vi "GetObjectConfigurationString.vi"(8 "ErrorIn":errorcluster, 10 "Label":string, 11 "ReferenceIn":refnum<class "AppConfigJSON.lvclass">) -> (0 "ErrorOut":errorcluster, 1 "String":string, 2 "Identification":string, 3 "ReferenceOut":refnum<class "AppConfigJSON.lvclass">)   [LabVIEW 2021, in "AppConfigJSON.lvclass"]
uses:
  AppConfigJSON.lvclass
  AppConfigJSON.lvclass/AppConfigJSON.ctl
  <vilib>/JDP Science/JSONtext/Config Files/Config File.lvclass
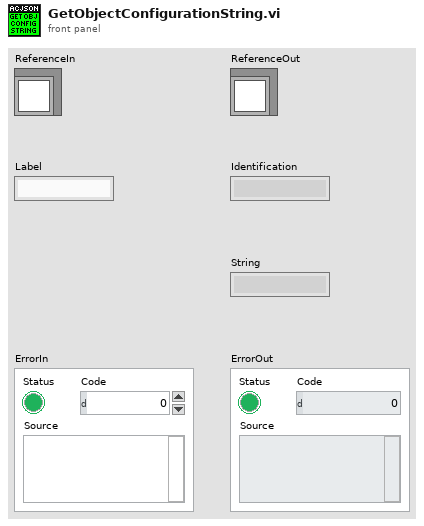
[diagram p1: front panel]
types:
  T1 = typedef "AppConfigJSON.lvclass/ObjectAttributes.ctl" = cluster{"Name":string, "ConfigFilePath":path, "Objects":T2[], "ApplicationBasePath":path, "ObjectName":string}
  T2 = typedef "IApplicationConfiguration.lvclass/ObjectDataDetails.ctl" = cluster{"ObjectName":string, "ObjectType":string, "Interfaces":T3[]}
  T3 = typedef "IApplicationConfiguration.lvclass/ObjectData.ctl" = cluster{"Label":string, "ObjectName":string, "Type":string}
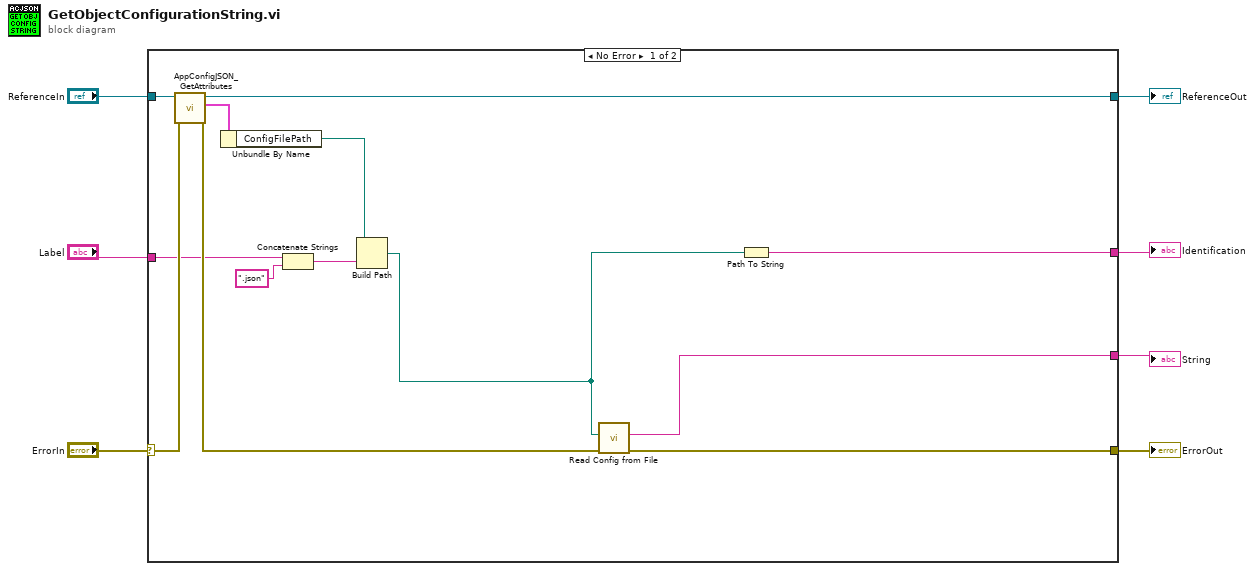
[diagram p0: block diagram]
diagram:
  n1 = case shown="No Error" "ErrorIn" {
    selector: "ErrorIn" -> [w19 w21]
    tunnel: [w18 w21] -> w6
    tunnel: [w15 w20] -> w4
    tunnel: "ReferenceIn" -> [w16 w20]
    tunnel: "Label" -> [w11 _]
    tunnel: [w10 _] -> w2
    tunnel: [w8 _] -> w1
    frame No Error {
      n2 = call "AppConfigJSON_GetAttributes.vi"("ErrorIn"=w19, "ReferenceIn"=w16) -> ("ErrorOut"=w18:errorcluster, "Data"=w17:T1, "ReferenceOut"=w15:refnum<class "AppConfigJSON.lvclass">)  [unwired: 6 in, 1 out]
      n3 = Unbundle By Name(w17) -> ("ConfigFilePath"=w12:path)
      n4 = Concatenate Strings(w11, ".json" ("string")) -> (w14:string)
      n5 = Build Path(base path=w12, name or relative path=w14) -> (appended path=w9:path)
      n6 = call <vilib>:"Read Config from File.vi"("error in (no error)"=w18, "config file path"=w9) -> ("<JSON>Config"=w10:string)  [unwired: 6 in, 3 out]
      n7 = Path To String(path=w9) -> (string=w8:string)
    }
    frame Error {
    }
  }
  "ErrorOut" <- w6
  "ReferenceOut" <- w4
  "String" <- w2
  "Identification" <- w1
